vi "Frequency Modulator 2.vi"(10 "Waveform In":waveform(dbl), 11 "Op. Frequency":dbl=100.0) -> (2 "Waveform Out":waveform(dbl), 3 "FFT - (Peak)":cluster{"f0":dbl, "df":dbl, "magnitude":dbl[]})   [LabVIEW 2014, in "Aquisicao de Dados.lvlib"]
uses:
  Aquisicao de Dados.lvlib
  <vilib>/Waveform/WDTOps.llb/WDT Number of Waveform Samples DBL.vi
  <vilib>/express/express analysis/Spectral/Block/exnSpectralBlock spectral measurements peak poly.vi
  <vilib>/express/express analysis/Spectral/Block/exnSpectralBlock spectral measurements peak WFM.vi
  <vilib>/express/express analysis/Spectral/XNode/ExpressSpectralMeasurementsBlockNode.xnode
  <vilib>/measure/NI_MABase.lvlib
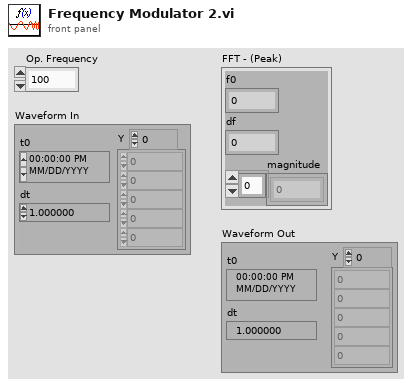
[diagram p1: front panel]
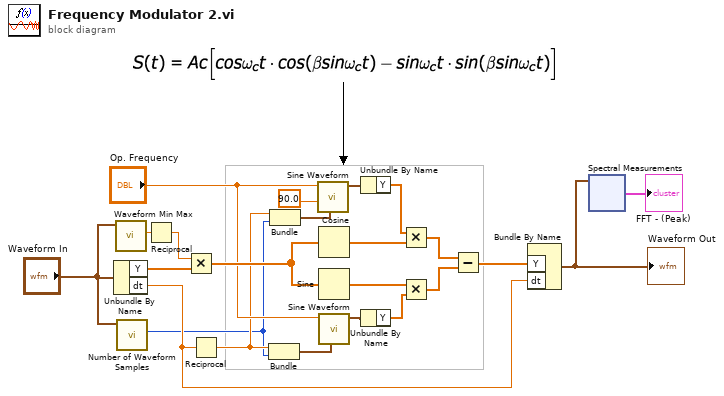
[diagram p0: block diagram]
diagram:
  n1 = Unbundle By Name("Waveform In") -> ("Y"=w7:dbl[], "dt"=w22:dbl)
  n2 = call <vilib>:"Waveform Min Max.vi"("waveform in"="Waveform In") -> ("Y max"=w5:dbl)  [unwired: 5 in, 5 out]
  n3 = call-poly <vilib>:"Number of Waveform Samples.vi"("waveform in"="Waveform In") -> ("number of samples"=w16:i32)  [unwired: 8 in, 2 out]
  n4 = Reciprocal(x=w5) -> (1/x=w6:dbl)
  n5 = Multiply(x=w6, y=w7) -> (x*y=w23:dbl[])
  n6 = Reciprocal(x=w22) -> (1/x=w17:dbl)
  n7 = Bundle(w17, "number of samples"=w16) -> (w11:cluster{dbl, "number of samples":i32})  [unwired: 1 in]
  n8 = Bundle(w17, "number of samples"=w16) -> (w10:cluster{dbl, "number of samples":i32})  [unwired: 1 in]
  n9 = call <vilib>:"Sine Waveform.vi"("sampling info"=w10, "phase"=90.0, "frequency"="Op. Frequency") -> ("signal out"=w19:waveform(dbl))  [unwired: 7 in, 1 out]
  n10 = Cosine(x=w23) -> (cos(x)=w1:dbl[])
  n11 = Sine(x=w23) -> (sin(x)=w2:dbl[])
  n12 = call <vilib>:"Sine Waveform.vi"("sampling info"=w11, "frequency"="Op. Frequency") -> ("signal out"=w18:waveform(dbl))  [unwired: 8 in, 1 out]
  n13 = Unbundle By Name(w19) -> ("Y"=w15:dbl[])
  n14 = Unbundle By Name(w18) -> ("Y"=w14:dbl[])
  n15 = Multiply(x=w15, y=w1) -> (x*y=w3:dbl[])
  n16 = Multiply(x=w2, y=w14) -> (x*y=w4:dbl[])
  n17 = Subtract(x=w3, y=w4) -> (x-y=w12:dbl[])
  n18 = Bundle By Name("Y"=w12, "dt"=w22) -> (w21:waveform(dbl))  [unwired: 1 in]
  "Waveform Out" <- w21
  n19 = xnode "Spectral Measurements"("Signals"=w21) -> ("FFT - (Peak)"=→"FFT - (Peak)":cluster{"f0":dbl, "df":dbl, "magnitude":dbl[]})  [unwired: 1 in, 2 out]
